vi "Create FP Item.vi"(6 "Cluster Component":bool, 8 "error in (no error)":errorcluster, 10 "GObject In":refnum<vi>, 11 "GString in":refnum<class "String.lvclass">) -> (0 "error out":errorcluster, 1 "Is Control":bool, 2 "Is Indicator":bool, 3 "GString out":refnum<class "String.lvclass">, 4 "All Objects Created":refnum<class "Object.lvclass">[](array[class]), 5 "Is Visible":bool)   [LabVIEW 2017, in "Front Panel Publisher.lvlib" / "String.lvclass"]
uses:
  String.lvclass
  Control_class/Control.lvclass
  Object_class/Object.lvclass
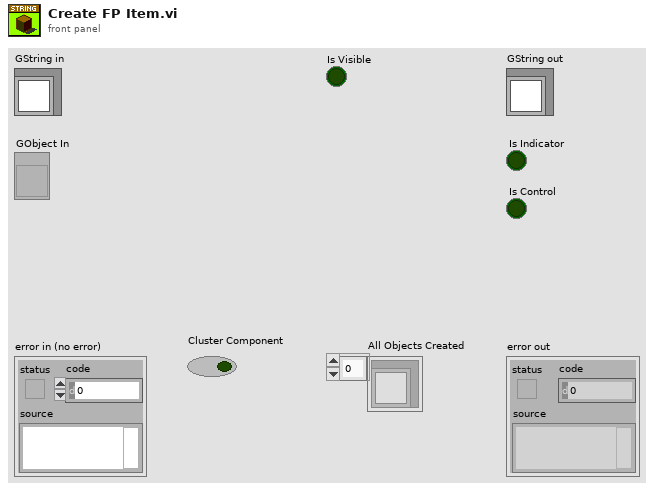
[diagram p1: front panel]
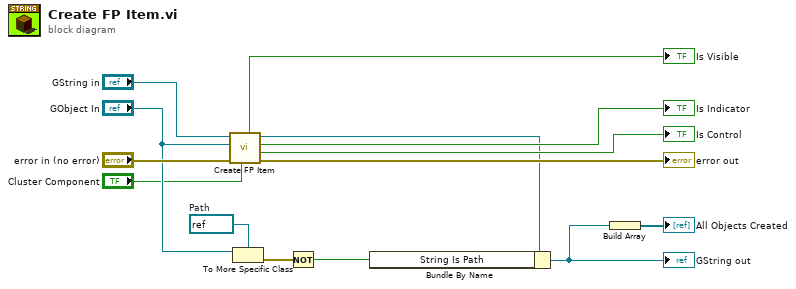
[diagram p0: block diagram]
diagram:
  w6 = refnum<vi> refnum  # Path
  n1 = call-parent "Create FP Item.vi"("Cluster Component"="Cluster Component", "error in (no error)"="error in (no error)", "GObject In"="GObject In", "GControl in"="GString in") -> ("error out"=→"error out":errorcluster, "Is Control"=→"Is Control":bool, "Is Indicator"=→"Is Indicator":bool, "GControl out"=w11:refnum<class "String.lvclass">, "Is Visible"=→"Is Visible":bool)  [unwired: 2 in, 1 out]
  n2 = To More Specific Class(target class=w6, reference="GObject In") -> (error out=w5:errorcluster)  [unwired: 1 in, 1 out]
  n3 = Not(x=w5) -> (.not. x?=w4:bool)
  n4 = Bundle By Name(cluster=w11, "String Is Path"=w4) -> (w3:refnum<class "String.lvclass">)
  "GString out" <- w3
  n5 = Build Array(w3) -> (→"All Objects Created":refnum<class "String.lvclass">[])
